vi "DSCProgClientEPICS Only.vi"() -> ()   [LabVIEW 2011]
uses:
  <vilib>/variable/tagger/epics/API/internal/List Records (By Ref).vi
  <vilib>/variable/tagger/epics/API/internal/Undeploy EPICS Client (By Ref).vi
  <vilib>/variable/tagger/epics/API/NI_EPICS_Client.lvlib
panel:
  out "error out":errorcluster
  out "error out 2":errorcluster
  out "records":string[](array[string])
  in  "stop":bool
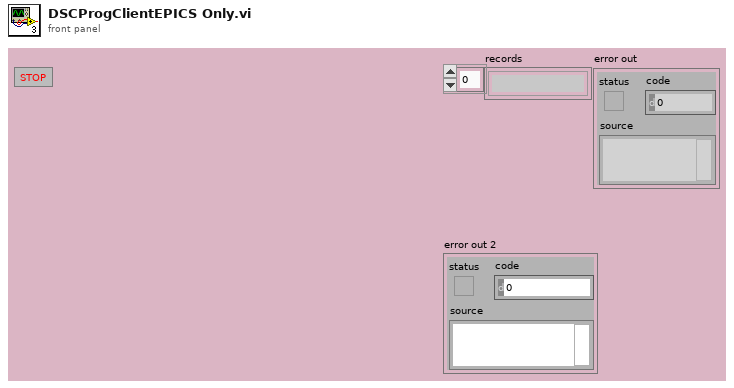
[diagram p1: front panel]
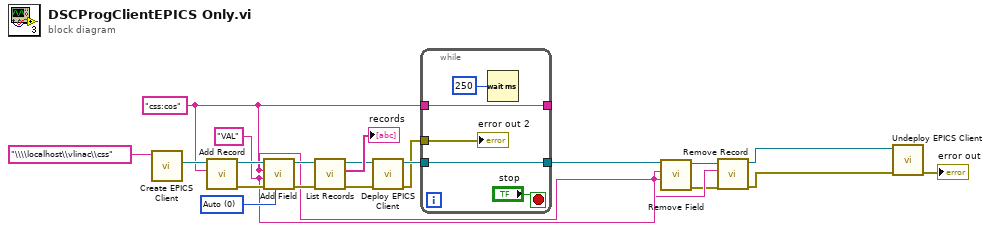
[diagram p0: block diagram]
diagram:
  w19 = u16 0 items=["Auto", "Double", "Bool", "String", "Short", "Float", "Enum", "Long", "Array of Double"] ("data type")
  w7 = "VAL" ("field name")
  w5 = "css:cos" ("record name")
  n1 = call <vilib>:"Create EPICS Client.vi"("EPICS Client URL in"="\\\\localhost\\vlinac\\css") -> ("EPICS Client ref"=w12:refnum<data-value>)  [unwired: 8 in, 2 out]
  n2 = call <vilib>:"Add Record.vi"("record name"=w5, "EPICS Client ref in"=w12) -> ("error out"=w10:errorcluster, "EPICS Client ref out"=w11:refnum<data-value>)  [unwired: 6 in, 2 out]
  n3 = call <vilib>:"Add Field.vi"("data type"=w19, "error in (no error)"=w10, "field name"=w7, "record name"=w5, "EPICS Client ref in"=w11) -> ("error out"=w18:errorcluster, "EPICS Client ref out"=w17:refnum<data-value>)  [unwired: 3 in, 2 out]
  n4 = call-poly <vilib>:"List Records.vi"("error in (no error)"=w18, "EPICS Client ref in"=w17) -> ("error out"=w14:errorcluster, "records"=→"records":string[], "EPICS Client ref out"=w15:refnum<data-value>)  [unwired: 7 in]
  n5 = call <vilib>:"Deploy EPICS Client.vi"("error in (no error)"=w14, "EPICS Client ref in"=w15) -> ("error out"=w9:errorcluster, "EPICS Client ref out"=w13:refnum<data-value>)  [unwired: 8 in]
  n6 = while {
    tunnel: w13 -> [w23]
    tunnel: [w23] -> w8
    tunnel: w5 -> [w22]
    tunnel: [w22] -> _
    tunnel: w9 -> [w21]
    stop <- "stop" stop-if-true
    n7 = Wait (ms)(milliseconds to wait=u32 250) -> ()  [unwired: 1 out]
    "error out 2" <- w21
  }
  n8 = call <vilib>:"Remove Field.vi"("record name"=w5, "field name"=w7, "EPICS Client ref in"=w8) -> ("error out"=w3:errorcluster, "EPICS Client ref out"=w6:refnum<data-value>)  [unwired: 7 in]
  n9 = call <vilib>:"Remove Record.vi"("error in (no error)"=w3, "record name"=w5, "EPICS Client ref in"=w6) -> ("error out"=w2:errorcluster, "EPICS Client ref out"=w4:refnum<data-value>)  [unwired: 7 in]
  n10 = call-poly <vilib>:"Undeploy EPICS Client.vi"("error in (no error)"=w2, "EPICS Client ref"=w4) -> ("error out"=→"error out":errorcluster)  [unwired: 9 in]
